vi "Read Intake Current.vi"(8 "Proposed Power":dbl, 11 "Current":dbl) -> (1 "Actual Power":dbl, 2 "Reverse Trip?":bool, 3 "Forward Trip?":bool)   [LabVIEW 2015]
uses:
  Common Code/Change Detect Boolean.vi
  Common Code/Utilities/TimeManager.vi
  Robot Global Data.vi
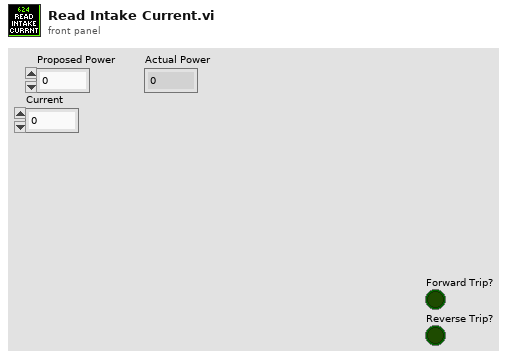
[diagram p1: front panel]
types:
  T1 = typedef "Dashboard Control Data.ctl" = cluster{"Shooter Presets":T2, "Encoder Control":T4, "Steer PID output":cluster{"output high":dbl, "output low":dbl}, " Steer PID gains":cluster{"proportional gain (Kc)":dbl, "integral time (Ti, min)":dbl, "derivative time (Td, min)":dbl}, "Drivetrain Settings":T5, "Vision Packet":T6, "Dashboard Drivetrain Command":T7, "Info/Command Cluster":T9, "Ball Vision Packet":T10, "Intake Presets":T12, "Intake Encoder Control":T14, "Climb Presets":T15, "Goal Output Range":cluster{"output high":dbl, "output low":dbl}, "Enabled Systems":T16, "Auton Presets":T17, "Pressure M":dbl, "Pressure B":dbl}
  T2 = typedef "Shooter Presets.ctl" = cluster{"Batter Shot":T3, "Deep Middle Shot":T3, "Manual Shot":T3, "Left Ticks Per Rotation":dbl, "Right Ticks Per Rotation":dbl, "Low Bar Shot":T3, "Shooter RPM Tolerance":dbl, "IIR Filter Power":dbl, "Trigger Power":dbl, "Fire from Load Delay":i32, "Max Angle":dbl, "Min Angle":dbl, "Angle PID gains":cluster{"P":dbl, "I":dbl, "D":dbl}, "Angle Output":cluster{"output high":dbl, "output low":dbl}, "Shooter Angle Tolerance":dbl, "Vision Shoot x^2":dbl, "Vision Shoot x":dbl, "Offset Angle":dbl, "High Goal Center Height":dbl, "Feed Forward Max Accel":dbl, "Feed Forward Kv":dbl, "Backwards Trigger":dbl, "Shot Finish Delay (ms)":dbl, "Angle Max Current":dbl, "Angle Current Trip Time":dbl, "Intake Angle":dbl, "Vision Shoot c":dbl, "Reset?":bool, "Servo Release Delay":dbl, "Servo Idle Angle":i32, "Servo Hold Angle":i32, "Angle Pot x":dbl, "Angle Pot c":dbl, "Ignore Angle?":bool, "Manual Output?":bool, "Manual Out":dbl, "Max RPM":dbl, "Safty Frist Angle":dbl, "Intake Danger Height":dbl, "Angle Pot B":i32, "Angle Pot M":dbl, "FF Finish RPM":dbl, "RPM PID Right":cluster{"P":dbl, "I":dbl, "D":dbl, "FF":dbl}, "RPM PID Left":cluster{"P":dbl, "I":dbl, "D":dbl, "FF":dbl}, "Backwards RPM":dbl, "Vision RPM":dbl}
  T3 = typedef "Shot Presets.ctl" = cluster{"Left":dbl, "Right":dbl, "Angle":dbl}
  T4 = typedef "Encoder Control.ctl" = cluster{"Right Tick Constant":dbl, "Left Tick Constant":dbl, "Reset?":bool, "Y Dist":cluster{"PID gains":cluster{"proportional gain (Kc)":dbl, "integral time (Ti, min)":dbl, "derivative time (Td, min)":dbl}}, "Y Stop Thresh":dbl, "Y Stop Speed":dbl}
  T5 = typedef "Drivetrain Settings.ctl" = cluster{"Gyro Tolerance":dbl, "Throttle Ramp (ms)":dbl, "Angular rate compensation":bool, "Throttle to Rate Scale":dbl, "Rate compensation gain":dbl, "Kv":dbl, "Ka":dbl, "Feed Forward P":dbl, "Feed Forward D":dbl, "Goal Vision PID gains":cluster{"proportional gain (Kc)":dbl, "integral time (Ti, min)":dbl, "derivative time (Td, min)":dbl}, "Goal Detection Window":dbl, "Creep Rate":dbl}
  T6 = typedef "Goal Vision Packet.ctl" = cluster{"Distance":dbl, "Center X":dbl, "Center Y":dbl, "Found Target?":bool, "Robot Center":dbl, "Angle":dbl}
  T7 = typedef "Dashboard Drivetrain Command.ctl" = cluster{"Drivetrain Vision":T8}
  T8 = typedef "Drivetrain Vision.ctl" = cluster{"Goal Window":dbl, "Ball Window":dbl}
  T9 = typedef "Ball Tracking Command Cluster.ctl" = cluster{"Distance to Ball":dbl, "Desired Angle":dbl, "Command":enum16{"Turn to Ball", "Turn to Angle", "Get Distance"}, "Pixels from Center":dbl}
  T10 = typedef "Ball Vision Packet.ctl" = cluster{"Ball Detected?":bool, "Distance to Ball":dbl, "Desired Angle":dbl, "Pixels from Center":dbl, "Tracking mode":T11}
  T11 = typedef "Tracking Mode.ctl" = enum16{"Turn to Ball", "Turn to Angle"}
  T12 = typedef "Intake Presets.ctl" = cluster{"Intake Speed":dbl, "Outake Speed":dbl, "Low Height":dbl, "Half Height":dbl, "Full Height":dbl, "Angle Speed":dbl, "Angle Tolerance":dbl, "Encoder Scale":dbl, "Load Height":dbl, "Output Range":T13, "Rotation Power Max/Min":dbl, "MaxCurrent":dbl, "Intake Trip Time":dbl, "Idle Height":dbl, "Max Height":dbl, "Reset Encoders?":bool, "PID gains":cluster{"proportional gain (Kc)":dbl, "integral time (Ti, min)":dbl, "derivative time (Td, min)":dbl}, "Intake Stop Delay":u32}
  T13 = typedef "Drivetrain Output Range.ctl" = cluster{"output high":dbl, "output low":dbl}
  T14 = typedef "IntakeEcoderControl.ctl" = cluster{"Arm Tick Constant":dbl, "Reset?":bool, "Y Dist":cluster{"PID gains":cluster{"proportional gain (Kc)":dbl, "integral time (Ti, min)":dbl, "derivative time (Td, min)":dbl}}, "Y Stop Thresh":dbl, "Y Stop Speed":dbl}
  T15 = typedef "Climb Presets.ctl" = cluster{"Pull Power":dbl, "Time to Hold":dbl, "Extend Power":dbl}
  T16 = typedef "Enabled Systems.ctl" = cluster{"Shoot":bool, "Intake":bool, "DT":bool, "Gyro":bool, "100ms":bool, "US":bool}
  T17 = typedef "Autonomous Presets.ctl" = cluster{"Pitch Limit":dbl, "Roll Limit":dbl, "Ultrasonic Limit":dbl, "Start Position":dbl, "Cross Position":dbl}
  T18 = typedef "WPI_DriverStationRobotMode2.ctl" = enum16{"Autonomous Disabled", "Autonomous Enabled", "Teleop Disabled", "Teleop Enabled", "Disconnected", "Finish", "Test Disabled", "Test Enabled", "Emergency Stopped"}
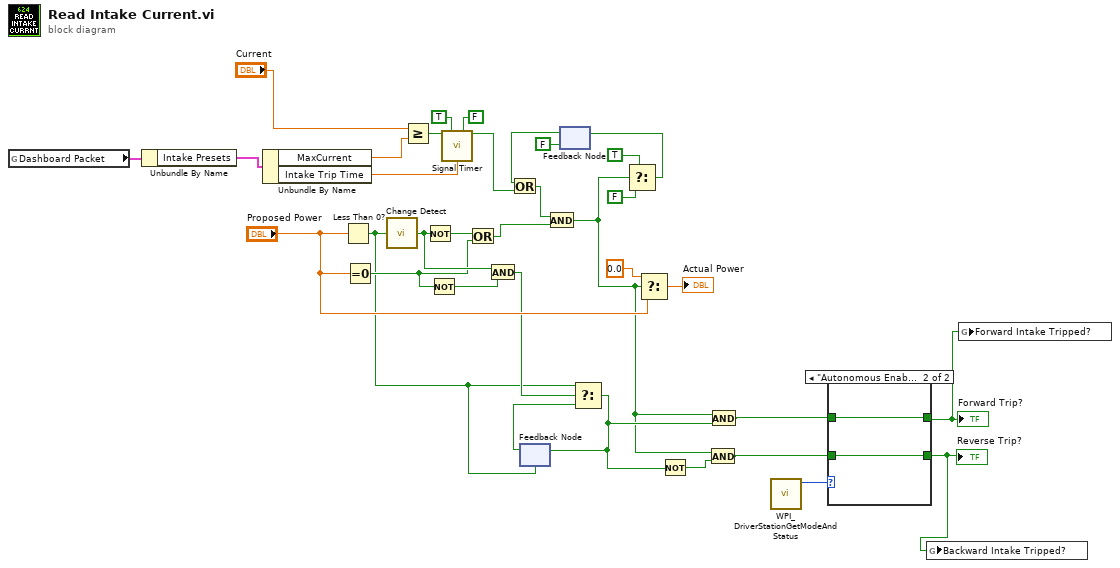
[diagram p0: block diagram]
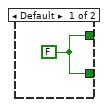
[diagram p2: hidden frame]
diagram:
  n1 = global read "Robot Global Data.vi" "Dashboard Packet"() -> (w34:T1)
  n2 = Unbundle By Name(w34) -> ("Intake Presets"=w33:T12)
  n3 = Unbundle By Name(w33) -> ("MaxCurrent"=w32:dbl, "Intake Trip Time"=w30:dbl)
  n4 = Less Than 0?(x="Proposed Power") -> (x < 0?=w8:bool)
  n5 = Equal To 0?(x="Proposed Power") -> (x = 0?=w10:bool)
  n6 = call-poly "Change Detect.vi"("In"=w8) -> ("Changed?"=w12:bool)
  n7 = Greater Or Equal?(x="Current", y=w32) -> (x >= y?=w31:bool)
  n8 = Not(x=w12) -> (.not. x?=w26:bool)
  n9 = Not(x=w10) -> (.not. x?=w11:bool)
  n10 = call "Signal Timer.vi"("Input"=w31, "Edge"=TRUE, "Interval"=w30, "Pull"=FALSE) -> ("Filtered Output"=w27:bool)  [unwired: 11 in]
  n11 = Or(x=w26, y=w10) -> (x .or. y?=w25:bool)
  n12 = And(x=w12, y=w11) -> (x .and. y?=w9:bool)
  n13 = feedback #1(w8) -> (w16:bool)
  n14 = feedback #2(FALSE) -> (w20:bool)
  n15 = Or(x=w20, y=w27) -> (x .or. y?=w24:bool)
  n16 = And(x=w24, y=w25) -> (x .and. y?=w13:bool)
  n17 = Select(t=w8, s=w9, f=w16) -> (s? t:f=w15:bool)
  n18 = feedback-in #1(w15) -> ()
  n19 = Select(t=TRUE, s=w13, f=FALSE) -> (s? t:f=w21:bool)
  n20 = feedback-in #2(w21) -> ()
  n21 = Select(t=0.0, s=w13, f="Proposed Power") -> (s? t:f=→"Actual Power":dbl)
  n22 = Not(x=w15) -> (.not. x?=w14:bool)
  n23 = And(x=w13, y=w14) -> (x .and. y?=w4:bool)
  n24 = And(x=w13, y=w15) -> (x .and. y?=w3:bool)
  n25 = call <vilib>:"WPI_DriverStationGetModeAndStatus.vi"() -> ("Robot Mode"=w5:T18)  [unwired: 10 in, 1 out]
  n26 = case shown="\"Autonomous Enabled\", \"Teleop Enabled\"" w5 {
    tunnel: [w35 w37] -> w2
    tunnel: w4 -> [_ w37]
    tunnel: [w35 w36] -> w1
    tunnel: w3 -> [_ w36]
    frame Default {
      w35 = FALSE
    }
    frame "Autonomous Enabled", "Teleop Enabled" {
    }
  }
  "Forward Trip?" <- w1
  "Reverse Trip?" <- w2
  n27 = global write "Robot Global Data.vi" "Backward Intake Tripped?"(w2) -> ()
  n28 = global write "Robot Global Data.vi" "Forward Intake Tripped?"(w1) -> ()
